vi "is_poly_vi.vi"   [LabVIEW 2015]
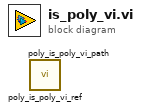
[diagram p0: block diagram]
diagram:
  n1 = call "poly_is_poly_vi_ref.vi"() -> ()  [unwired: 9 in, 1 out]
  n2 = call "poly_is_poly_vi_path.vi"() -> ()  [unwired: 9 in, 1 out]
